vi "pf_Camera_Control_manager.vi"(7 "Action":T3=enum."Get", 8 "error in (no error)":errorcluster, 10 "Camera Control in":T1={"Port Name"="", "Port Number"=-1, "IMAQ Session"=refnum, "PeakDetector_Mode"=enum."2D only", "Window.W"=0, "Window.H"=0}, 11 "IMAQ Session in":refnum<k11>) -> (0 "error out":errorcluster, 2 "Camera Control out":T1={"Port Name"="", "Port Number"=-1, "IMAQ Session"=refnum, "PeakDetector_Mode"=enum."2D only", "Window.W"=0, "Window.H"=0}, 3 "IMAQ Session out":refnum<k11>)   [LabVIEW 2025, in "Photonfocus_Toolkit.lvlib"]
doc: "manages all the parameters needed by the library."
uses:
  Photonfocus_Toolkit.lvlib
  Controls/pf_Camera_ctrl_mngr_action.ctl
  Controls/pf_Camera_Control.ctl
  Controls/pf_PeakDetector_Mode.ctl
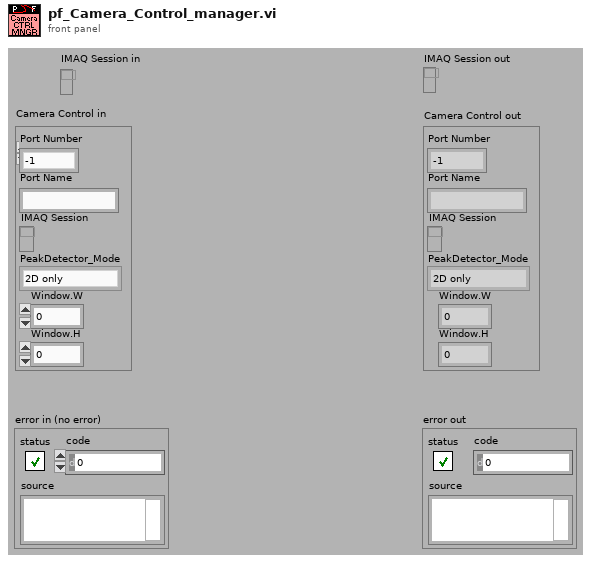
[diagram p1: front panel]
types:
  T1 = typedef "Photonfocus_Toolkit.lvlib/pf_Camera_Control.ctl" = cluster{"Port Name":string, "Port Number":i32, "IMAQ Session":refnum<k11>, "PeakDetector_Mode":T2, "Window.W":u32, "Window.H":u32}
  T2 = typedef "Photonfocus_Toolkit.lvlib/pf_PeakDetector_Mode.ctl" = enum16{"Undefined", "2D only", "2D and 3D", "3D only"}
  T3 = typedef "Photonfocus_Toolkit.lvlib/pf_Camera_ctrl_mngr_action.ctl" = enum16{"Create", "Destroy", "Set", "Get"}
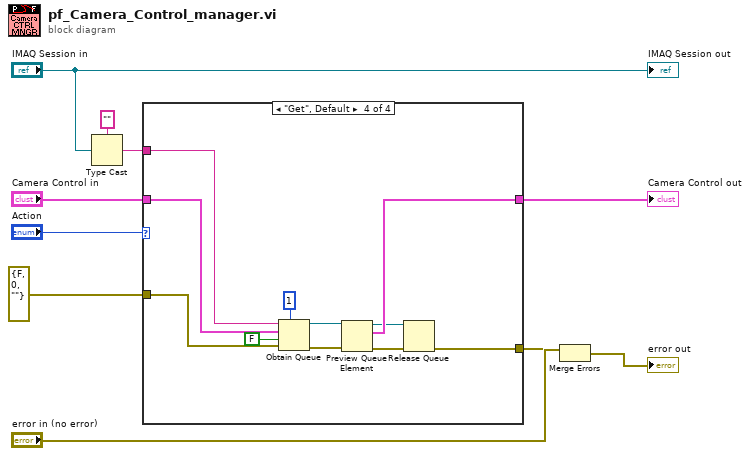
[diagram p0: block diagram]
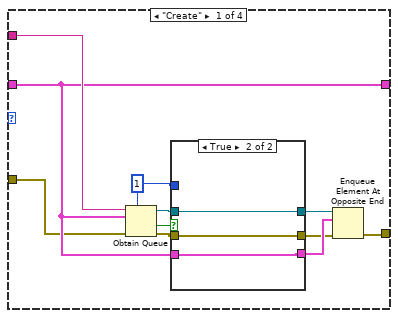
[diagram p2: hidden frame]
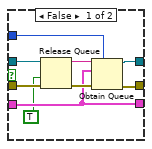
[diagram p3: hidden frame]
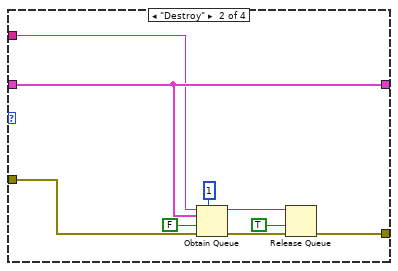
[diagram p4: hidden frame]
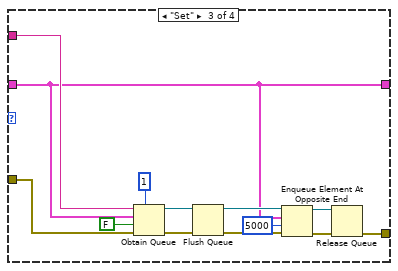
[diagram p5: hidden frame]
diagram:
  n1 = Type Cast(type="", x="IMAQ Session in") -> (*(type *) &x=w1:string)
  n2 = case shown="\"Get\", Default" "Action" {
    tunnel: [w17 w35 w44 w57] -> w7
    tunnel: [w12 w38 w48 w62] -> w4
    tunnel: "Camera Control in" -> [w12 w38 w48 w60]
    tunnel: w1 -> [w13 w34 w49 w61]
    tunnel: errorcluster {"status"=FALSE, "code"=0, "source"=""} ("error in (no error)") -> [w11 w36 w46 w59]
    frame "Create" {
      w16 = 1 ("max queue size (-1, unlimited)")
      n3 = Obtain Queue(max queue size (-1, unlimited)=w16, name (unnamed)=w13, element data type=w12, error in (no error)=w11) -> (queue out=w15:refnum<queue>, created new?=w14:bool, error out=w18:errorcluster)  [unwired: 1 in]
      n4 = case shown="True" w14 {
        tunnel: w18 -> [w30 w33]
        tunnel: [w25 w33] -> w19
        tunnel: w15 -> [w29 w32]
        tunnel: w16 -> [w26 _]
        tunnel: w12 -> [w23 w31]
        tunnel: [w24 w32] -> w20
        tunnel: [w23 w31] -> w21
        frame False {
          n5 = Release Queue(queue=w29, force destroy? (F)=TRUE, error in (no error)=w30) -> (queue name=w27:string, error out=w28:errorcluster)  [unwired: 1 out]
          n6 = Obtain Queue(max queue size (-1, unlimited)=w26, name (unnamed)=w27, element data type=w23, error in (no error)=w28) -> (queue out=w24:refnum<queue>, error out=w25:errorcluster)  [unwired: 1 in, 1 out]
        }
        frame True {
        }
      }
      n7 = Enqueue Element At Opposite End(queue=w20, element=w21, error in (no error)=w19) -> (error out=w17:errorcluster)  [unwired: 3 out]
    }
    frame "Destroy" {
      n8 = Obtain Queue(max queue size (-1, unlimited)=1, name (unnamed)=w34, element data type=w38, create if not found? (T)=FALSE, error in (no error)=w36) -> (queue out=w39:refnum<queue>, error out=w42:errorcluster)  [unwired: 1 out]
      n9 = Release Queue(queue=w39, force destroy? (F)=TRUE, error in (no error)=w42) -> (error out=w35:errorcluster)  [unwired: 2 out]
    }
    frame "Set" {
      n10 = Obtain Queue(max queue size (-1, unlimited)=1, name (unnamed)=w49, element data type=w48, create if not found? (T)=FALSE, error in (no error)=w46) -> (queue out=w52:refnum<queue>, error out=w53:errorcluster)  [unwired: 1 out]
      n11 = Flush Queue(queue=w52, error in (no error)=w53) -> (queue out=w51:refnum<queue>, error out=w50:errorcluster)  [unwired: 1 out]
      n12 = Enqueue Element At Opposite End(queue=w51, element=w48, timeout in ms (-1)=5000, error in (no error)=w50) -> (queue out=w43:refnum<queue>, error out=w45:errorcluster)  [unwired: 1 out]
      n13 = Release Queue(queue=w43, error in (no error)=w45) -> (error out=w44:errorcluster)  [unwired: 3 out]
    }
    frame "Get", Default {
      n14 = Obtain Queue(max queue size (-1, unlimited)=1, name (unnamed)=w61, element data type=w60, create if not found? (T)=FALSE, error in (no error)=w59) -> (queue out=w64:refnum<queue>, error out=w66:errorcluster)  [unwired: 1 out]
      n15 = Preview Queue Element(queue=w64, error in (no error)=w66) -> (queue out=w56:refnum<queue>, element=w62:T1, error out=w58:errorcluster)  [unwired: 2 out]
      n16 = Release Queue(queue=w56, error in (no error)=w58) -> (error out=w57:errorcluster)  [unwired: 3 out]
    }
  }
  "Camera Control out" <- w4
  n17 = Merge Errors("error in (no error)", w7) -> (→"error out":errorcluster)
  "IMAQ Session out" <- "IMAQ Session in"
